vi "SlippyInterval.vi"(3 "Reset":bool, 5 "Interval (ms)":i32) -> (0 "Next Interval (ms)":i32, 1 "Elapsed Time (ms)":u32, 2 "Slip Count":i32)   [LabVIEW 2020]
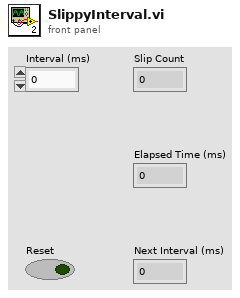
[diagram p1: front panel]
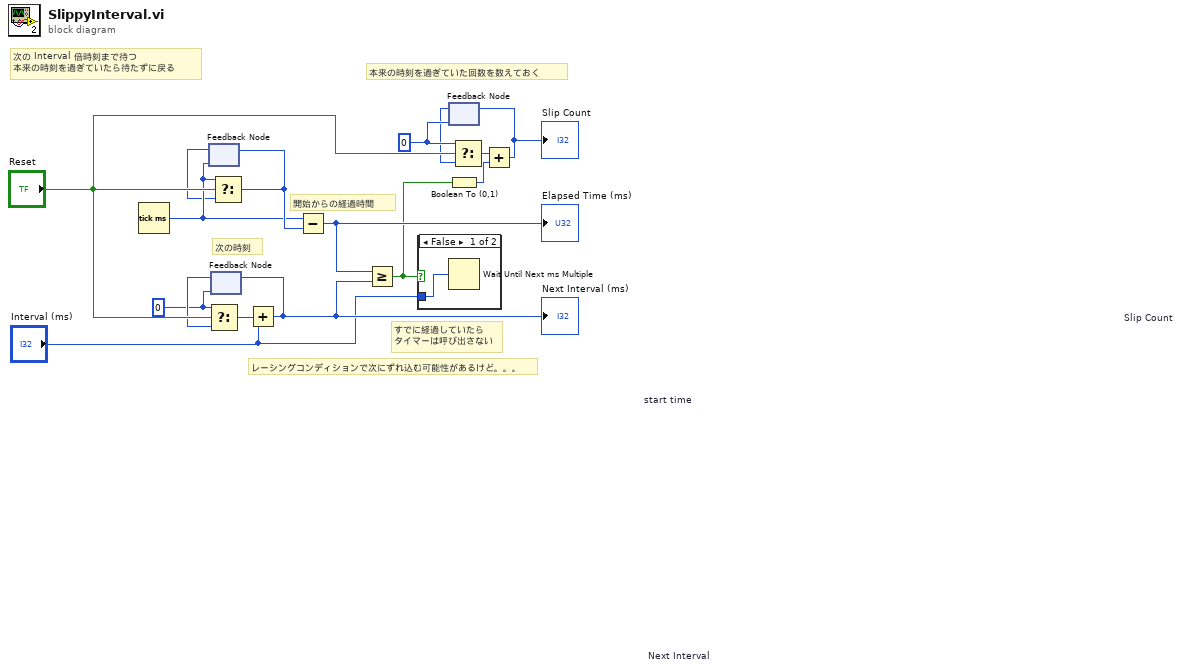
[diagram p0: block diagram]
diagram:
  w9 = 0
  w4 = 0
  # "次の Interval 倍時刻まで待つ\n本来の時刻を過ぎていたら待たずに戻る"
  # "本来の時刻を過ぎていた回数を数えておく"
  # "レーシングコンディションで次にずれ込む可能性があるけど。。。"
  # "すでに経過していたら\nタイマーは呼び出さない"
  # "次の時刻"
  # "開始からの経過時間"
  n1 = Tick Count (ms)() -> (millisecond timer value=w2:u32)
  n2 = feedback #1 "start time"(w2) -> (w1:u32)
  n3 = feedback #2 "Next Interval"(w4) -> (w5:i32)
  n4 = Select(t=w4, s="Reset", f=w5) -> (s? t:f=w6:i32)
  n5 = Select(t=w2, s="Reset", f=w1) -> (s? t:f=w3:u32)
  n6 = feedback-in #1(w3) -> ()
  n7 = Add(x=w6, y="Interval (ms)") -> (x+y=w16:i32)
  "Next Interval (ms)" <- w16
  n8 = feedback-in #2(w16) -> ()
  n9 = Subtract(x=w2, y=w3) -> (x-y=w15:u32)
  "Elapsed Time (ms)" <- w15
  n10 = Greater Or Equal?(x=w15, y=w16) -> (x >= y?=w10:bool)
  n11 = case shown="False" w10 {
    tunnel: "Interval (ms)" -> [w17 _]
    frame False {
      n12 = Wait Until Next ms Multiple(millisecond multiple=w17) -> ()  [unwired: 1 out]
    }
    frame True {
    }
  }
  n13 = feedback #3 "Slip Count"(w9) -> (w8:i32)
  n14 = Boolean To (0,1)(Boolean=w10) -> (0, 1=w12:i16)
  n15 = Select(t=w9, s="Reset", f=w8) -> (s? t:f=w11:i32)
  n16 = Add(x=w11, y=w12) -> (x+y=w13:i32)
  "Slip Count" <- w13
  n17 = feedback-in #3(w13) -> ()
